vi "Untitled 1 (SubVI).vi"(9 "c":dbl, 10 "b":dbl, 11 "a":dbl) -> (3 "D":dbl)   [LabVIEW 2016]
uses:
  <vilib>/express/express arith-compare/Formula/XNode/ExpressFormulaBlockNode.xnode
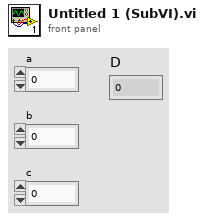
[diagram p1: front panel]
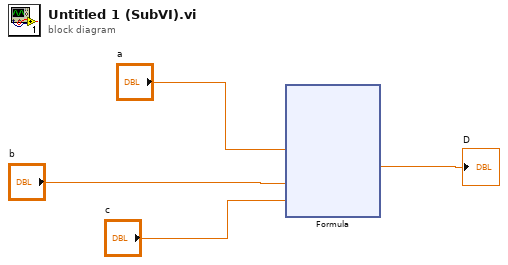
[diagram p0: block diagram]
diagram:
  n1 = xnode "Formula"("a"="a", "b"="b", "c"="c") -> ("Result"=→"D":dbl)  [unwired: 1 in, 1 out]
